vi "Test Enqueue Message VIs.vi"() -> ()   [LabVIEW 2013]
doc: "This Continuous Measurement sample project is based on the Queued Message Handler template.\n\nThe Event Handling Loop generates messages based on user interface actions.\n\nThe Message Handling Loop processes messages generated by the Event Handling Loop, or by other messages. There are also Acquisition and Logging message handling loop subVIs, and a chart updating loop."
uses:
  <vilib>/Utility/error.llb/DialogType.ctl
  support/Message Queue/Message Cluster.ctl
  <userlib>/_OpenG.lib/appcontrol/appcontrol.llb/ClassID Names Enum__ogtk.ctl
  support/Message Queue/Enqueue Message (Single).vi
  <vilib>/Utility/error.llb/Error Cluster From Error Code.vi
  <userlib>/_OpenG.lib/array/array.llb/Search 1D Array (I32)__ogtk.vi
  <userlib>/_OpenG.lib/array/array.llb/Index 1D Array Elements (Variant)__ogtk.vi
  support/Message Queue/Enqueue Message (Array).vi
  support/Message Queue/Enqueue Message (MultiLine String w Array).vi
  <vilib>/ErrorRing/Error Ring.xnode
  support/User Event - Stop/User Event - Stop.lvlib
  support/Message Queue/Message Queue.lvlib
panel:
  in  "Test to Run":u16(ring) items=["", "Test Single Message", "Test Multiple Messages Single String", "Test Multiple Messages Array of Strings", "Test Single Message with String Argument", "Test Single Message with Message Data", "Test Mutiple Messages Single String with String Arguments", "Test Multiple Messages Single String with Message Data", "Test Mutiple Messages String Array with String Arguments", "Test Mutiple Messages String Array with Message Data", "Test Mutiple Messages Separate Enqueue Calls", "Test Priority Enqueue Single Message", "Test Priority Enqueue Multiple Messages Single String", "Test Priority Enqueue Multiple Messages String Array", "Test Priority Enqueue Multiple Messages Single String with Message Data", "Test Priority Enqueue Multiple Messages String Array with Message Data", "Test Error Handler"]
  out "Status":string
  in  "Exit":bool
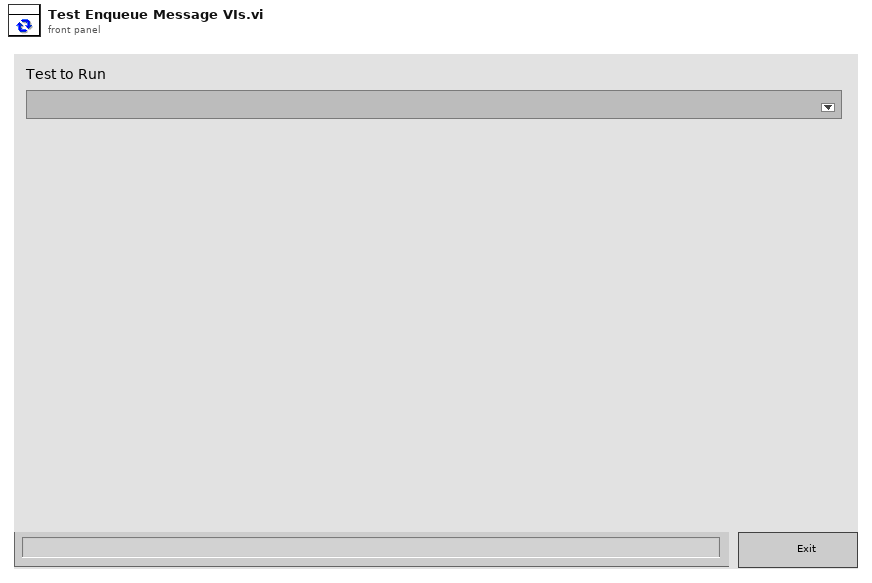
[diagram p1: front panel]
types:
  T1 = cluster{"Macro:Initialize":string, "Macro:Exit":string, "Core":cluster{"Current VI Reference":refnum<vi>, "Close Panel on Exit?":bool}}
  T2 = typedef "Message Queue.lvlib/All Message Queues.ctl" = cluster{"UI":refnum<queue>, "Acquisition":refnum<queue>, "Logging":refnum<queue>}
  T3 = enum32{"invalid app kind", "Development System", "Run Time System", "Student Edition", "Embedded LabVIEW", "Evaluation", "Custom"}
  T4 = typedef "Message Queue.lvlib/Message Cluster.ctl" = cluster{"Message":string, "Message Data":variant}
  T5 = typedef "ClassID Names Enum__ogtk.ctl" = enum32{"0 <undefined>", "1 <undefined>", "2 <undefined>", "Generic", "Decoration", "Text", "Control", "ColorBox", "Boolean", "RefNum", "Variant", "Path", "ListBox", "Table", "Array", "Picture", "ActiveXContainer", "Numeric", "Digital", "NamedNumeric", "ColorRamp", "Slide", "GraphOrChart", "WaveformChart", "WaveformGraph", "IntensityChart", "IntensityGraph", "String", "IOName", "ComboBox", "Cluster", "Panel", "Knob", "NumWithScale", "Ring", "Enum", "GObject", "Plot", "Cursor", "NumericText", "Scale", "ColorScale", "GraphScale", "ColorGraphScale", "TypedRefNum", "OldKnobScale", "MCListbox", "MeasureData", "BVTag", "DAQName", "VISAName", "IVIName", "SlideScale", "TabControl", "Page", "TabArrayTabControl", "ConPane"}
  T6 = enum32{"Invalid", "Standard", "Closed", "Hidden", "Minimized", "Maximized"}
  T7 = typedef "DialogType.ctl" = u16
  T8 = cluster{"element":T4, "error constant":errorcluster}
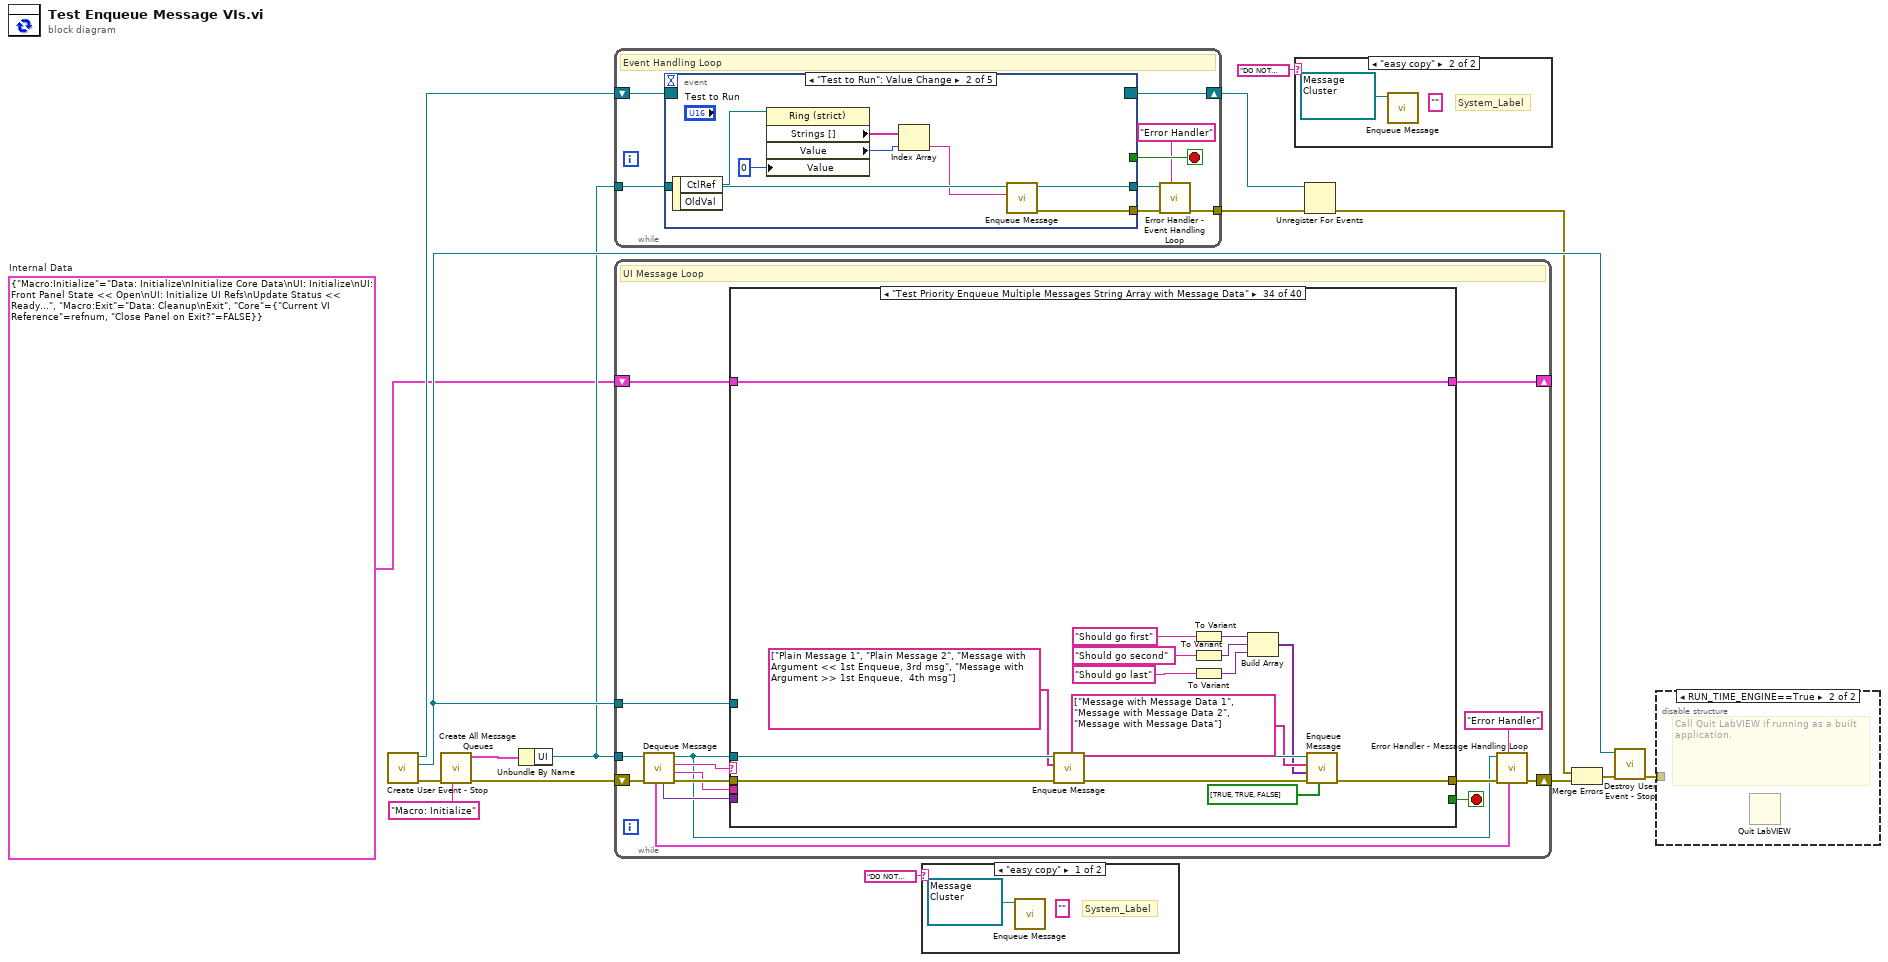
[diagram p0: block diagram]
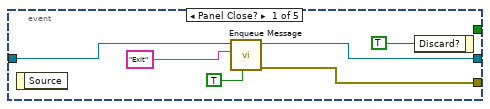
[diagram p5: hidden frame]
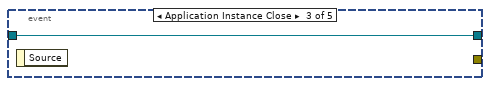
[diagram p6: hidden frame]
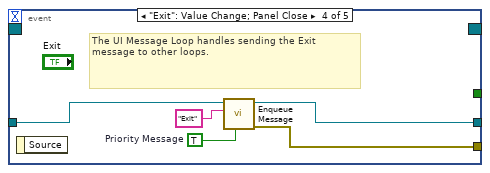
[diagram p7: hidden frame]
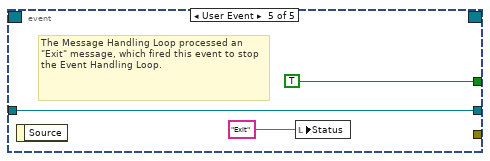
[diagram p8: hidden frame]
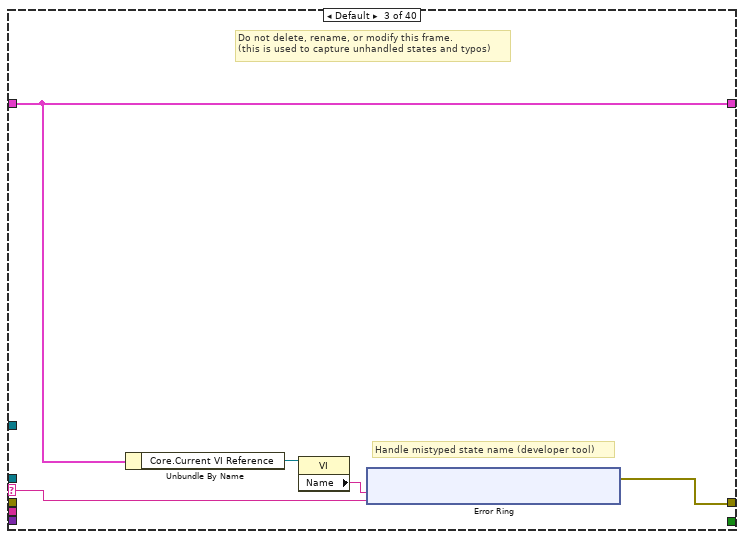
[diagram p11: hidden frame]
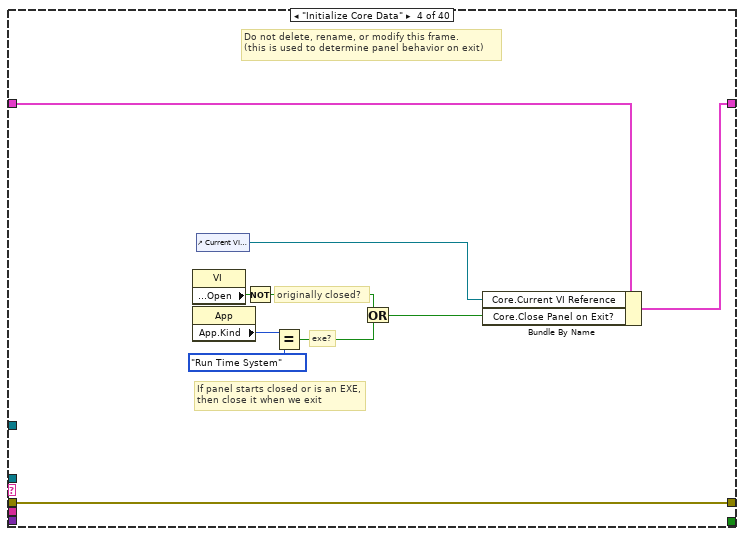
[diagram p12: hidden frame]
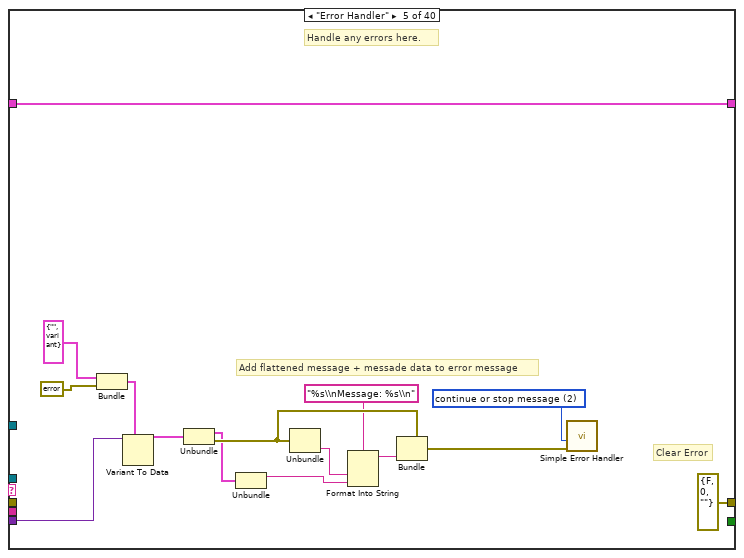
[diagram p13: hidden frame]
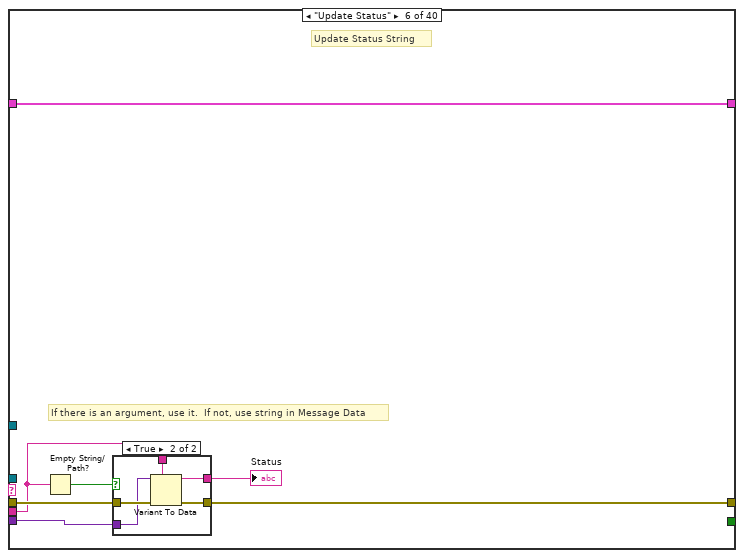
[diagram p14: hidden frame]
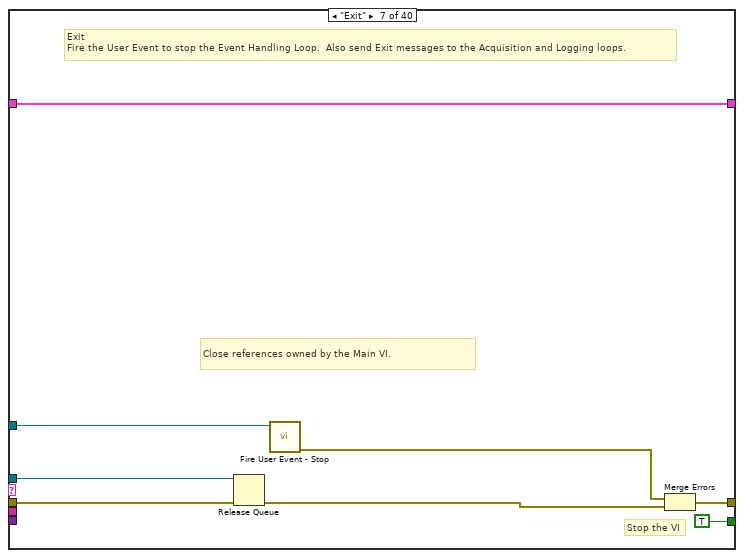
[diagram p16: hidden frame]
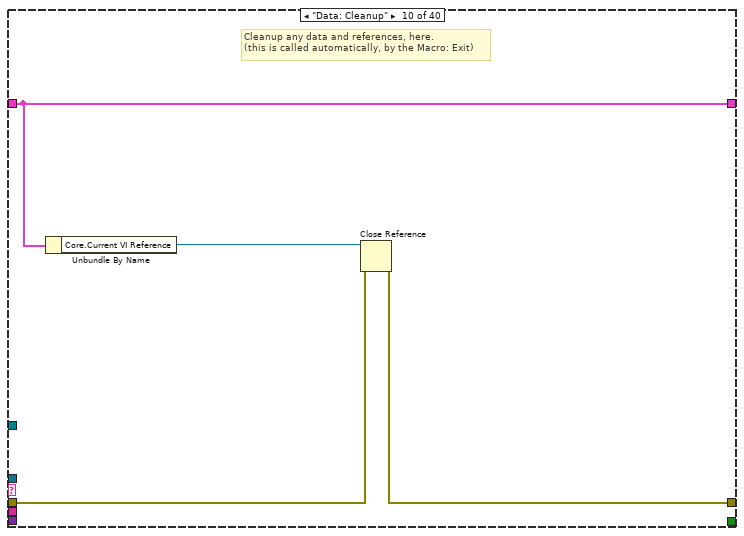
[diagram p19: hidden frame]
diagram:
  w4 = T1 {"Macro:Initialize"="Data: Initialize\nInitialize Core Data\nUI: Initialize\nUI: Front Panel State << Open\nUI: Initialize UI Refs\nUpdate Status << Ready...", "Macro:Exit"="Data: Cleanup\nExit", "Core"={"Current VI Reference"=refnum, "Close Panel on Exit?"=FALSE}}  # Internal Data
  n1 = call "Create User Event - Stop.vi"() -> ("error out"=w12:errorcluster, "User Event - Stop"=w13:refnum<user-event>, "Stop Event Registration Refnum"=w14:refnum<event-registration>)  [unwired: 9 in]
  n2 = call "Create All Message Queues.vi"("Message"="Macro: Initialize", "error in (no error)"=w12) -> ("error out"=w10:errorcluster, "Message Queues out"=w11:T2)  [unwired: 8 in]
  n3 = Unbundle By Name(w11) -> ("UI"=w7:refnum<queue>)
  n4 = while {
    tunnel: w7 -> [w23]
    tunnel: [w20] -> w15
    shift-right: [w22] -> w8
    shift-left: w14 -> [w24]
    stop <- w21 stop-if-true
    # "Event Handling Loop"
    n5 = event shown="[1] \"Test to Run\": Value Change" {
      selector: w24 -> [_ _ _ _ _]
      dyn-events: [_ _ _ _ _] -> w22
      timeout: _ -> [_ _ _ _ _]
      tunnel: [_ _ _ _ TRUE ("Discard?")] -> w21
      tunnel: w23 -> [w28 w38 w39 w41 w45]
      tunnel: [w26 w36 _ w44 _] -> w19
      tunnel: [w27 w37 w39 w40 w45] -> w18
      event Panel Close? {
        n6 = event-data() -> ()  [unwired: 1 in, 1 out]
        n7 = call-poly "Enqueue Message.vi"("Priority Message? (F)"=TRUE, "Message"="Exit", "Message Queue"=w28) -> ("error out"=w26:errorcluster, "dup Message Queue"=w27:refnum<queue>)  [unwired: 7 in]
        n8 = event-data("Discard?"=TRUE) -> ()  [unwired: 1 in, 1 out]
      }
      event "Test to Run": Value Change {
        n9 = event-data() -> ("CtlRef"=w35:refnum<vi>)  [unwired: 1 in, 1 out]
        n10 = property class="Ring (strict)"(reference=w35, "Value"=u16 0) -> ("Strings []"=w34:string[], "Value"=w33:u16)  [unwired: 1 in, 2 out]
        n11 = Index Array(array=w34, index=w33) -> (element=w32:string)
        n12 = call-poly "Enqueue Message.vi"("Message"=w32, "Message Queue"=w38) -> ("error out"=w36:errorcluster, "dup Message Queue"=w37:refnum<queue>)  [unwired: 8 in]
      }
      event Application Instance Close {
        n13 = event-data() -> ()  [unwired: 1 in, 1 out]
      }
      event "Exit": Value Change; Panel Close {
        w42 = TRUE  # Priority Message
        # "The UI Message Loop handles sending the Exit message to other loops."
        n14 = event-data() -> ()  [unwired: 1 in, 1 out]
        n15 = call-poly "Enqueue Message.vi"("Priority Message? (F)"=w42, "Message"="Exit", "Message Queue"=w41) -> ("error out"=w44:errorcluster, "dup Message Queue"=w40:refnum<queue>)  [unwired: 7 in]
      }
      event User Event {
        # "The Message Handling Loop processed an \"Exit\" message, which fired this event to stop the Event Handling Loop."
        n16 = event-data() -> ()  [unwired: 1 in, 1 out]
        n17 = local write "Status"("Exit" ("Exit String")) -> ()
      }
    }
    n18 = call "Error Handler - Event Handling Loop.vi"("Error Handler Message"="Error Handler" ("Message"), "error in (no error)"=w19, "Message Queue"=w18) -> ("dup error in"=w20:errorcluster)  [unwired: 7 in, 1 out]
  }
  n19 = while {
    tunnel: w7 -> [w61]
    tunnel: w13 -> [w57]
    shift-right: [w60] -> w16
    shift-left: w10 -> [w62]
    shift-right: [w51] -> _
    shift-left: w4 -> [w52]
    stop <- w56 stop-if-true
    # "UI Message Loop"
    n20 = call "Dequeue Message.vi"("error in (no error)"=w62, "Message Queue"=w61) -> ("error out"=w59:errorcluster, "Argument"=w54:string, "Message"=w58:string, "dup Message Queue"=w50:refnum<queue>, "Message Data"=w53:variant, "element"=w48:T4)  [unwired: 4 in]
    n21 = case shown="\"Test Priority Enqueue Multiple Messages String Array with Message Data\"" w58 {
      selector: w58 -> [_ _ w68 _ _ _ _ _ _ _ _ _ _ _ _ _ _ _ _ _ _ _ _ _ _ _ _ _ _ _ _ _ _ _ _ _ _ w379 w389 w401]
      tunnel: w54 -> [_ _ _ _ _ w106 _ _ _ _ _ _ _ w157 w165 _ _ _ _ _ _ _ _ _ _ _ _ _ _ _ _ _ _ _ _ _ _ _ w387 _]
      tunnel: [w64 w66 w67 w89 errorcluster {"status"=FALSE, "code"=0, "source"=""} ("error out") w108 w123 w128 w129 w132 w136 w146 w155 w158 w167 w192 w195 w198 w212 w215 w220 w225 w230 w236 w241 w252 w257 w272 w291 w300 w309 w318 w334 w350 w353 w367 w376 w377 w384 w394] -> w55
      tunnel: w59 -> [w64 w66 _ w89 _ w110 w121 w128 w129 w133 w136 w146 w155 w159 w168 w192 w197 w207 w212 w216 w221 w226 w231 w237 w242 w253 w258 w273 w278 w298 w307 w316 w332 w348 w355 w367 w376 w378 w385 w399]
      tunnel: [_ _ _ _ _ _ TRUE _ _ _ _ _ _ _ _ _ _ _ _ _ _ _ _ _ _ _ _ _ _ _ _ _ _ _ _ _ _ _ _ _] -> w56
      tunnel: w57 -> [_ _ _ _ _ _ w122 _ _ _ _ _ _ _ _ _ _ _ _ _ _ _ _ _ _ _ _ _ _ _ _ _ _ _ _ _ _ _ _ _]
      tunnel: w53 -> [_ _ _ _ w103 w109 _ _ _ _ _ _ _ _ _ _ _ _ _ _ _ _ _ _ _ _ _ _ _ _ _ _ _ _ _ _ _ _ _ w398]
      tunnel: w52 -> [w63 w65 w70 w81 w104 w111 w125 w127 w130 w131 w135 w142 w154 w156 w164 w191 w193 w201 w211 w217 w222 w227 w232 w238 w243 w254 w259 w274 w292 w301 w310 w319 w335 w351 w357 w363 w375 w380 w390 w402]
      tunnel: [w63 w65 w70 w80 w104 w111 w125 w127 w130 w131 w135 w142 w154 w156 w164 w191 w193 w201 w211 w217 w222 w227 w232 w238 w243 w254 w259 w274 w292 w301 w310 w319 w335 w351 w357 w363 w375 w380 w390 w402] -> w51
      tunnel: w50 -> [_ _ _ _ _ _ w120 _ _ _ _ _ _ _ _ _ w196 w206 _ w214 w219 w224 w229 w235 w240 w251 w256 w271 w279 w299 w308 w317 w333 w349 w356 _ _ _ _ _]
      frame "", "Idle" {
        # "Executes when the state queue is empty\nAlso commented out messages"
      }
      frame "---------- Core ----------" {
        # "Do not put any code in this frame.\n(it is a separator no-op)"
      }
      frame Default {
        # "Handle mistyped state name (developer tool)"
        # "Do not delete, rename, or modify this frame.\n(this is used to capture unhandled states and typos)"
        n22 = Unbundle By Name(w70) -> ("Core.Current VI Reference"=w69:refnum<vi>)
        n23 = property class="VI"(reference=w69) -> ("Name"=w71:string)  [unwired: 1 in, 2 out]
        n24 = xnode "Error Ring"("parameter 0"=w71, "parameter 1"=w68) -> ("error out"=w67:errorcluster)
      }
      frame "Initialize Core Data" {
        # "Do not delete, rename, or modify this frame.\n(this is used to determine panel behavior on exit)"
        # "originally closed?"
        # "exe?"
        # "If panel starts closed or is an EXE, then close it when we exit"
        n25 = property class="VI"() -> ("Front Panel.Open"=w88:bool)  [unwired: 2 in, 2 out]
        n26 = property class="App"() -> ("App.Kind"=w87:T3)  [unwired: 2 in, 2 out]
        n27 = control-ref of="Current VI Reference"() -> (w82:refnum<vi>)
        n28 = Not(x=w88) -> (.not. x?=w85:bool)
        n29 = Equal?(x=w87, y=T3."Run Time System" ("Application:Kind")) -> (x = y?=w84:bool)
        n30 = Or(x=w85, y=w84) -> (x .or. y?=w83:bool)
        n31 = Bundle By Name(cluster=w81, "Core.Current VI Reference"=w82, "Core.Close Panel on Exit?"=w83) -> (w80:T1)
      }
      frame "Error Handler" {
        w102 = T7 2 items=["no dialog", "OK message", "continue or stop message", "OK message + warnings", "continue/stop + warnings"] ("type of dialog (OK msg:1)")
        # "Add flattened message + messade data to error message"
        # "Clear Error"
        # "Handle any errors here."
        n32 = Bundle("element"=T4 {"Message"="", "Message Data"=variant}, "error constant"=errorcluster {"status"=FALSE, "code"=0, "source"=""}) -> (w98:T8)  [unwired: 1 in]
        n33 = Variant To Data(type=w98, Variant=w103) -> (data=w97:T8)  [unwired: 1 in, 1 out]
        n34 = Unbundle(w97) -> ("element"=w94:T4, "error constant"=w96:errorcluster)
        n35 = Unbundle(w94) -> ("Message"=w92:string)  [unwired: 1 out]
        n36 = Unbundle(w96) -> ("source"=w91:string)  [unwired: 2 out]
        n37 = Format Into String(format string="%s\\nMessage: %s\\n", w91, w92) -> (resulting string=w93:string)  [unwired: 2 in, 1 out]
        n38 = Bundle(cluster=w96, "source"=w93) -> (w95:errorcluster)  [unwired: 2 in]
        n39 = call <vilib>:"Simple Error Handler.vi"("type of dialog (OK msg:1)"=w102, "error in (no error)"=w95) -> ()  [unwired: 3 in, 5 out]
      }
      frame "Update Status" {
        # "If there is an argument, use it.  If not, use string in Message Data"
        # "Update Status String"
        n40 = Empty String/Path?(string/path=w106) -> (empty?=w107:bool)
        n41 = case shown="True" w107 {
          tunnel: w110 -> [w112 w118]
          tunnel: w109 -> [_ w117]
          tunnel: w106 -> [w113 w116]
          tunnel: [w112 w115] -> w108
          tunnel: [w113 w114] -> w105
          frame False {
          }
          frame True {
            n42 = Variant To Data(error in=w118, type=w116, Variant=w117) -> (data=w114:string, error out=w115:errorcluster)
          }
        }
        "Status" <- w105
      }
      frame "Exit" {
        # "Close references owned by the Main VI."
        # "Stop the VI"
        # "Exit\nFire the User Event to stop the Event Handling Loop.  Also send Exit messages to the Acquisition and Logging loops."
        n43 = Release Queue(queue=w120, error in (no error)=w121) -> (error out=w119:errorcluster)  [unwired: 1 in, 2 out]
        n44 = call "Fire User Event - Stop.vi"("User Event - Stop"=w122) -> ("error out"=w124:errorcluster)  [unwired: 10 in]
        n45 = Merge Errors(w124, w119) -> (w123:errorcluster)
      }
      frame "---------- Data ----------" {
        # "Do not put any code in this frame.\n(It is a separator no-op. You can make a copy of this frame to create a new Data frame)"
      }
      frame "Data: Initialize" {
        # "Initialize the shift-register data, here.\n(data names are defined by what you wire into the bundle function)"
      }
      frame "Data: Cleanup" {
        # "Cleanup any data and references, here.\n(this is called automatically, by the Macro: Exit)"
        n46 = Unbundle By Name(w131) -> ("Core.Current VI Reference"=w134:refnum<vi>)
        n47 = Close Reference(reference=w134, error in (no error)=w133) -> (error out=w132:errorcluster)
      }
      frame "---------- UI ----------" {
        # "Do not put any code in this frame.\n(It is a separator no-op. You can make a copy of this frame to create a new UI frame)"
      }
      frame "UI: Initialize" {
        w137 = refnum<vi> refnum  # Boolean
        # "Initialize the User Interface, here.\n(this is called automatically, by the Macro: Init)"
        n48 = Unbundle By Name(w142) -> ("Core.Current VI Reference"=w145:refnum<vi>)
        n49 = call <userlib>:"MGI Get VI Control Ref[].vi"("VI (Caller)"=w145) -> ("Control Type[i]"=w144:T5[], "Control[i]"=w139:refnum<vi>[])  [unwired: 7 in, 2 out]
        n50 = call-poly <userlib>:"Search Array__ogtk.vi"("Array"=w144, "Element Data"=ClassID_Names_Enum__ogtk."Boolean" ("ClassID Name")) -> ("Indices of Elements"=w141:i32[])  [unwired: 7 in]
        n51 = call-poly <userlib>:"Index Array Elements__ogtk.vi"("indices"=w141, "array"=w139) -> ("elements"=w140:variant[])  [unwired: 9 in]
        n52 = Index Array(array=w139) -> (element=w138:refnum<vi>)  [unwired: 1 in]
        n53 = for {
          tunnel: w140 -> [w153] mode=indexing
          tunnel: w138 -> [w152]
          tunnel: w137 -> [w149]
          n54 = Variant To Data(type=w152, Variant=w153) -> (data=w151:refnum<vi>, error out=w150:errorcluster)  [unwired: 1 in]
          n55 = To More Specific Class(target class=w149, reference=w151, error in=w150) -> (specific class reference=w148:refnum<vi>)  [unwired: 1 out]
          n56 = property class="Bool"(reference=w148, "Value"=FALSE) -> ()  [unwired: 1 in, 2 out]
        }
      }
      frame "UI: Initialize UI Refs" {
        # "Package and Init UI Refs as Required"
      }
      frame "UI: Cursor Set" {
        # "Argument"
        # "Set and Unset Cursor Busy.\n(Usage: \"UI: Cursor Set >> Busy|Idle\")"
        n57 = case shown="\"Idle\", Default" w157 {
          tunnel: w159 -> [w161 w163]
          tunnel: [w160 w162] -> w158
          frame "Idle", Default {
            n58 = call <vilib>:"Unset Busy.vi"("error in (no error)"=w161) -> ("error out"=w160:errorcluster)  [unwired: 10 in]
          }
          frame "Busy" {
            n59 = call <vilib>:"Set Busy.vi"("error in (no error)"=w163) -> ("error out"=w162:errorcluster)  [unwired: 9 in, 1 out]
          }
        }
      }
      frame "UI: Front Panel State" {
        # "Argument"
        # "Set Front Panel Open or Closed\n(Usage: \"UI: Front Panel State >> Open|Close\")"
        n60 = Unbundle By Name(w164) -> ("Core.Current VI Reference"=w166:refnum<vi>)
        n61 = case shown="\"Open\", Default" w165 {
          tunnel: w168 -> [w172 w185]
          tunnel: [w174 w186] -> w167
          tunnel: w166 -> [w173 w183]
          frame "Open", Default {
            n62 = property class="VI"(reference=w173, error in=w172) -> (reference out=w170:refnum<vi>, error out=w171:errorcluster, "Front Panel.Open"=w169:bool)
            n63 = case shown="True" w169 {
              tunnel: [w177 w180] -> w174
              tunnel: w171 -> [w176 w180]
              tunnel: w170 -> [w175 _]
              frame False {
                n64 = invoke class="VI" method="FP.Open"(reference=w175, error in=w176, "Activate"=TRUE, "State"=T6."Standard") -> (error out=w177:errorcluster)  [unwired: 1 in, 4 out]
              }
              frame True {
              }
            }
          }
          frame "Close" {
            n65 = property class="VI"(reference=w183, error in=w185) -> (reference out=w182:refnum<vi>, error out=w184:errorcluster, "Front Panel.Open"=w181:bool)
            n66 = case shown="True" w181 {
              tunnel: [w187 w190] -> w186
              tunnel: w184 -> [w187 w189]
              tunnel: w182 -> [_ w188]
              frame False {
              }
              frame True {
                n67 = invoke class="VI" method="FP.Close"(reference=w188, error in=w189) -> (error out=w190:errorcluster)  [unwired: 1 in, 2 out]
              }
            }
          }
        }
      }
      frame "---------- Macro ----------" {
        # "Do not put any code in this frame.\n(It is a separator no-op. You can make a copy of this frame to create a new Macro frame)"
      }
      frame "Macro: Initialize" {
        # "Initialization Macro\n(This is called once, when the VI starts)"
        n68 = Unbundle By Name(w193) -> ("Macro:Initialize"=w194:string)
        n69 = call-poly "Enqueue Message.vi"("error in (no error)"=w197, "Message"=w194, "Message Queue"=w196) -> ("error out"=w195:errorcluster)  [unwired: 7 in, 1 out]
      }
      frame "Macro: Exit" {
        # "Exit Macro\n(This is called once, when the VI exits)"
        n70 = Unbundle By Name(w201) -> ("Core.Close Panel on Exit?"=w210:bool)
        n71 = Unbundle By Name(w201) -> ("Macro:Exit"=w200:string)
        n72 = Select(t="UI: Front Panel State >> Close", s=w210, f="") -> (s? t:f=w205:string)
        n73 = call-poly "Enqueue Message.vi"("Priority Message? (F)"=TRUE, "error in (no error)"=w207, "Message"=w205, "Message Queue"=w206) -> ("error out"=w202:errorcluster, "dup Message Queue"=w203:refnum<queue>)  [unwired: 6 in]
        n74 = call-poly "Enqueue Message.vi"("Priority Message? (F)"=FALSE, "error in (no error)"=w202, "Message"=w200, "Message Queue"=w203) -> ("error out"=w198:errorcluster)  [unwired: 6 in, 1 out]
      }
      frame "---------- Tests ----------" {
        # "Template Separator\n(You can make a copy of, or modify, this frame)"
      }
      frame "Test Single Message" {
        # "Test Single Message\nTest Single String Message without Argument or Message Data"
        n75 = call-poly "Enqueue Message.vi"("error in (no error)"=w216, "Message"="Plain Message 1", "Message Queue"=w214) -> ("error out"=w215:errorcluster)  [unwired: 7 in, 1 out]
      }
      frame "Test Multiple Messages Single String" {
        # "Test Multiple Messages Single String\nTest Multiple Messages Single String without Argument or Message Data"
        n76 = call-poly "Enqueue Message.vi"("error in (no error)"=w221, "Message"="Plain Message 1\nPlain Message 2", "Message Queue"=w219) -> ("error out"=w220:errorcluster)  [unwired: 7 in, 1 out]
      }
      frame "Test Multiple Messages Array of Strings" {
        # "Test Multiple Messages Array of Strings\nTest Multiple Messages Array of Strings without Argument or Message Data"
        n77 = call-poly "Enqueue Message.vi"("error in (no error)"=w226, "Message Array"=string[] ["Plain Message 1", "Plain Message 2"], "Message Queue"=w224) -> ("error out"=w225:errorcluster)  [unwired: 7 in, 1 out]
      }
      frame "Test Single Message with String Argument" {
        n78 = call-poly "Enqueue Message.vi"("error in (no error)"=w231, "Message"="Message with Argument << I Do NOT Agree", "Message Queue"=w229) -> ("error out"=w230:errorcluster)  [unwired: 7 in, 1 out]
      }
      frame "Test Single Message with Message Data" {
        n79 = call-poly "Enqueue Message.vi"("error in (no error)"=w237, "Message Data"="Data was on Star Trek?" ("Message"), "Message"="Message with Message Data", "Message Queue"=w235) -> ("error out"=w236:errorcluster)  [unwired: 6 in, 1 out]
      }
      frame "Test Mutiple Messages with String Arguments" {
        n80 = call-poly "Enqueue Message.vi"("error in (no error)"=w242, "Message"="Plain Message 1\nPlain Message 2\nMessage with Argument << 3rd msg arg\nMessage with Argument >> 4th msg arg", "Message Queue"=w240) -> ("error out"=w241:errorcluster)  [unwired: 7 in, 1 out]
      }
      frame "Test Multiple Messages Single String with Message Data" {
        w245 = variant ("Variant")
        n81 = To Variant(anything="3rd msg arg" ("Message")) -> (Variant=w248:variant)
        n82 = To Variant(anything="4th msg arg" ("Message")) -> (Variant=w247:variant)
        n83 = Build Array(w245, w245, w248, w247) -> (w244:variant[])
        n84 = call-poly "Enqueue Message.vi"("error in (no error)"=w253, "Message Data Array"=w244, "Message"="Plain Message 1\nPlain Message 2\nMessage with Message Data\nMessage with Message Data", "Message Queue"=w251) -> ("error out"=w252:errorcluster)  [unwired: 6 in, 1 out]
      }
      frame "Test Mutiple Messages String Array with String Arguments" {
        n85 = call-poly "Enqueue Message.vi"("error in (no error)"=w258, "Message Array"=string[] ["Plain Message 1", "Plain Message 2", "Message with Argument << 3rd msg", "Message with Argument >> 4th msg"], "Message Queue"=w256) -> ("error out"=w257:errorcluster)  [unwired: 7 in, 1 out]
      }
      frame "Test Mutiple Messages String Array with Message Data" {
        w266 = variant ("Variant")
        n86 = To Variant(anything="3rd msg arg" ("Message")) -> (Variant=w269:variant)
        n87 = To Variant(anything="4th msg arg" ("Message")) -> (Variant=w268:variant)
        n88 = Build Array(w266, w266, w269, w268) -> (w265:variant[])
        n89 = Initialize Array("Message with Message Data" ("Message"), 2 ("dimension size")) -> (w261:string[])
        n90 = Build Array (concatenate)(string[] ["Plain Message 1", "Plain Message 2"], w261) -> (w260:string[])
        n91 = call-poly "Enqueue Message.vi"("error in (no error)"=w273, "Message Data Array"=w265, "Message Array"=w260, "Message Queue"=w271) -> ("error out"=w272:errorcluster)  [unwired: 6 in, 1 out]
      }
      frame "Test Mutiple Messages Separate Enqueue Calls" {
        w286 = variant ("Variant")
        n92 = call-poly "Enqueue Message.vi"("error in (no error)"=w278, "Message Array"=string[] ["Plain Message 1", "Plain Message 2", "Message with Argument << 1st Enqueue, 3rd msg", "Message with Argument >> 1st Enqueue,  4th msg"], "Message Queue"=w279) -> ("error out"=w277:errorcluster, "dup Message Queue"=w276:refnum<queue>)  [unwired: 7 in]
        n93 = To Variant(anything="2nd Enqueue, 3rd msg arg" ("Message")) -> (Variant=w289:variant)
        n94 = To Variant(anything="2nd Enqueue, 4th msg arg" ("Message")) -> (Variant=w288:variant)
        n95 = Build Array(w286, w286, w289, w288) -> (w285:variant[])
        n96 = Initialize Array("Message with Message Data" ("Message"), 2 ("dimension size")) -> (w281:string[])
        n97 = Build Array (concatenate)(string[] ["Plain Message 1", "Plain Message 2"], w281) -> (w280:string[])
        n98 = call-poly "Enqueue Message.vi"("error in (no error)"=w277, "Message Data Array"=w285, "Message Array"=w280, "Message Queue"=w276) -> ("error out"=w291:errorcluster)  [unwired: 6 in, 1 out]
      }
      frame "Test Priority Enqueue Single Message" {
        # "Should see Priority Single Message message first"
        n99 = call-poly "Enqueue Message.vi"("error in (no error)"=w298, "Message Array"=string[] ["Plain Message 1", "Plain Message 2", "Message with Argument << 1st Enqueue, 3rd msg", "Message with Argument >> 1st Enqueue,  4th msg"], "Message Queue"=w299) -> ("error out"=w297:errorcluster, "dup Message Queue"=w296:refnum<queue>)  [unwired: 7 in]
        n100 = call-poly "Enqueue Message.vi"("Priority Message? (F)"=TRUE, "error in (no error)"=w297, "Message"="Priority Single Message", "Message Queue"=w296) -> ("error out"=w300:errorcluster)  [unwired: 6 in, 1 out]
      }
      frame "Test Priority Enqueue Multiple Messages Single String" {
        n101 = call-poly "Enqueue Message.vi"("error in (no error)"=w307, "Message Array"=string[] ["Plain Message 1", "Plain Message 2", "Message with Argument << 1st Enqueue, 3rd msg", "Message with Argument >> 1st Enqueue,  4th msg"], "Message Queue"=w308) -> ("error out"=w306:errorcluster, "dup Message Queue"=w305:refnum<queue>)  [unwired: 7 in]
        n102 = call-poly "Enqueue Message.vi"("Priority Message? (F)"=TRUE, "error in (no error)"=w306, "Message"="Message with Argument << Should go first\nMessage with Argument >> Should go second", "Message Queue"=w305) -> ("error out"=w309:errorcluster)  [unwired: 6 in, 1 out]
      }
      frame "Test Priority Enqueue Multiple Messages String Array" {
        n103 = call-poly "Enqueue Message.vi"("error in (no error)"=w316, "Message Array"=string[] ["Plain Message 1", "Plain Message 2", "Message with Argument << 1st Enqueue, 3rd msg", "Message with Argument >> 1st Enqueue,  4th msg"], "Message Queue"=w317) -> ("error out"=w315:errorcluster, "dup Message Queue"=w313:refnum<queue>)  [unwired: 7 in]
        n104 = call-poly "Enqueue Message.vi"("Priority Message? Array"=bool[] [TRUE, TRUE, FALSE], "error in (no error)"=w315, "Message Array"=string[] ["Message with Argument 1 << Should go first", "Message with Argument 2 >> Should go second", "Message with Argument << Should go last"], "Message Queue"=w313) -> ("error out"=w318:errorcluster)  [unwired: 6 in, 1 out]
      }
      frame "Test Priority Enqueue Multiple Messages Single String with Message Data" {
        n105 = call-poly "Enqueue Message.vi"("error in (no error)"=w332, "Message Array"=string[] ["Plain Message 1", "Plain Message 2", "Message with Argument << 1st Enqueue, 3rd msg", "Message with Argument >> 1st Enqueue,  4th msg"], "Message Queue"=w333) -> ("error out"=w331:errorcluster, "dup Message Queue"=w329:refnum<queue>)  [unwired: 7 in]
        n106 = To Variant(anything="Should go first" ("Message")) -> (Variant=w326:variant)
        n107 = To Variant(anything="Should go second" ("Message")) -> (Variant=w325:variant)
        n108 = To Variant(anything="Should go last" ("Message")) -> (Variant=w320:variant)
        n109 = Build Array(w326, w325, w320) -> (w323:variant[])
        n110 = call-poly "Enqueue Message.vi"("Priority Message? Array"=bool[] [TRUE, TRUE, FALSE], "error in (no error)"=w331, "Message Data Array"=w323, "Message"="Message with Message Data 1\nMessage with Message Data 2\nMessage with Message Data", "Message Queue"=w329) -> ("error out"=w334:errorcluster)  [unwired: 5 in, 1 out]
      }
      frame "Test Priority Enqueue Multiple Messages String Array with Message Data" {
        n111 = call-poly "Enqueue Message.vi"("error in (no error)"=w348, "Message Array"=string[] ["Plain Message 1", "Plain Message 2", "Message with Argument << 1st Enqueue, 3rd msg", "Message with Argument >> 1st Enqueue,  4th msg"], "Message Queue"=w349) -> ("error out"=w347:errorcluster, "dup Message Queue"=w345:refnum<queue>)  [unwired: 7 in]
        n112 = To Variant(anything="Should go first" ("Message")) -> (Variant=w341:variant)
        n113 = To Variant(anything="Should go second" ("Message")) -> (Variant=w340:variant)
        n114 = To Variant(anything="Should go last" ("Message")) -> (Variant=w337:variant)
        n115 = Build Array(w341, w340, w337) -> (w336:variant[])
        n116 = call-poly "Enqueue Message.vi"("Priority Message? Array"=bool[] [TRUE, TRUE, FALSE], "error in (no error)"=w347, "Message Data Array"=w336, "Message Array"=string[] ["Message with Message Data 1", "Message with Message Data 2", "Message with Message Data"], "Message Queue"=w345) -> ("error out"=w350:errorcluster)  [unwired: 5 in, 1 out]
      }
      frame "Test Error Handler" {
        # "This should be a string, not a number"
        n117 = call-poly "Enqueue Message.vi"("error in (no error)"=w355, "Message Data"=0, "Message"="Message with Message Data", "Message Queue"=w356) -> ("error out"=w353:errorcluster)  [unwired: 6 in, 1 out]
      }
      frame "Set All Test Buttons False" {
        w358 = refnum<vi> refnum  # Boolean
        n118 = Unbundle By Name(w363) -> ("Core.Current VI Reference"=w366:refnum<vi>)
        n119 = call <userlib>:"MGI Get VI Control Ref[].vi"("VI (Caller)"=w366) -> ("Control Type[i]"=w365:T5[], "Control[i]"=w360:refnum<vi>[])  [unwired: 7 in, 2 out]
        n120 = call-poly <userlib>:"Search Array__ogtk.vi"("Array"=w365, "Element Data"=ClassID_Names_Enum__ogtk."Boolean" ("ClassID Name")) -> ("Indices of Elements"=w362:i32[])  [unwired: 7 in]
        n121 = call-poly <userlib>:"Index Array Elements__ogtk.vi"("indices"=w362, "array"=w360) -> ("elements"=w361:variant[])  [unwired: 9 in]
        n122 = Index Array(array=w360) -> (element=w359:refnum<vi>)  [unwired: 1 in]
        n123 = for {
          tunnel: w361 -> [w374] mode=indexing
          tunnel: w359 -> [w373]
          tunnel: w358 -> [w370]
          n124 = Variant To Data(type=w373, Variant=w374) -> (data=w372:refnum<vi>, error out=w371:errorcluster)  [unwired: 1 in]
          n125 = To More Specific Class(target class=w370, reference=w372, error in=w371) -> (specific class reference=w369:refnum<vi>)  [unwired: 1 out]
          n126 = property class="Bool"(reference=w369, "Value"=FALSE) -> ()  [unwired: 1 in, 2 out]
        }
      }
      frame "---------- Messages ----------" {
        # "Template Separator\n(You can make a copy of, or modify, this frame)"
      }
      frame "Plain Message 1", "Plain Message 2", "Priority Single Message" {
        n127 = case shown="No Error" w378 {
          selector: w378 -> [w381 w383]
          tunnel: w379 -> [w382 _]
          tunnel: [w381 w383] -> w377
          frame No Error {
            n128 = One Button Dialog(message=w382) -> ()  [unwired: 1 in, 1 out]
          }
          frame Error {
          }
        }
      }
      frame "Message with Argument", "Message with Argument 1", "Message with Argument 2" {
        n129 = Concatenate Strings(w389, ", Argument = " ("string"), w387) -> (w386:string)
        n130 = case shown="No Error" w385 {
          selector: w385 -> [w391 w393]
          tunnel: w386 -> [w392 _]
          tunnel: [w391 w393] -> w384
          frame No Error {
            n131 = One Button Dialog(message=w392) -> ()  [unwired: 1 in, 1 out]
          }
          frame Error {
          }
        }
      }
      frame "Message with Message Data", "Message with Message Data 1", "Message with Message Data 2" {
        w397 = ", Message Data = " ("string")
        n132 = Variant To Data(error in=w399, type=w397, Variant=w398) -> (data=w396:string, error out=w395:errorcluster)
        n133 = Concatenate Strings(w401, w397, w396) -> (w400:string)
        n134 = case shown="No Error" w395 {
          selector: w395 -> [w403 w405]
          tunnel: w400 -> [w404 _]
          tunnel: [w403 w405] -> w394
          frame No Error {
            n135 = One Button Dialog(message=w404) -> ()  [unwired: 1 in, 1 out]
          }
          frame Error {
          }
        }
      }
    }
    n136 = call "Error Handler - Message Handling Loop.vi"("element"=w48, "Error Handler Message"="Error Handler" ("Message"), "error in (no error)"=w55, "Message Queue"=w50) -> ("dup error in"=w60:errorcluster)  [unwired: 6 in, 1 out]
  }
  n137 = case shown="\"easy copy\"" "DO NOT RUN!!" {
    frame "easy copy" {
      (unwired) "" ("Message")
      # "System_Label"
      n138 = call-poly "Enqueue Message.vi"("Message Queue"=refnum<queue> refnum) -> ()  [unwired: 9 in, 2 out]
    }
    frame Default {
    }
  }
  n139 = case shown="\"easy copy\"" "DO NOT RUN!!" {
    frame Default {
    }
    frame "easy copy" {
      (unwired) "" ("Message")
      # "System_Label"
      n140 = call-poly "Enqueue Message.vi"("Message Queue"=refnum<queue> refnum) -> ()  [unwired: 9 in, 2 out]
    }
  }
  n141 = Unregister For Events(event registration refnum=w8, error in=w15) -> (error out=w9:errorcluster)
  n142 = Merge Errors(w9, w16) -> (w5:errorcluster)
  n143 = call "Destroy User Event - Stop.vi"("error in (no error)"=w5, "User Event - Stop"=w13) -> ("error out"=w6:errorcluster)  [unwired: 9 in]
  n144 = disable-structure shown="RUN_TIME_ENGINE==True" {
    disable-tunnel: w6 -> [_ _]
    frame condition #0 (active) {
    }
    frame condition #1 {
      # "Call Quit LabVIEW if running as a built application."
      n145 = Quit LabVIEW() -> ()  [unwired: 1 in]
    }
  }
